vi "Mod_OFDM_Generate_Frame_per_Sub_Carrier.vi"(0 "Configure Variant":variant, 7 "Pool of Modulators":T3, 11 "error in":errorcluster, 12 "Pool of Data Sources":T2 {"Register Initial State" format="%08x"}, 13 "Symbol names in Frame":string[](array[string]), 14 "# of Symbols":i32) -> (4 "Parameters per OFDM Symbol":T1 {"Data Source"."Data Source"."Register Initial State" format="%08x"}, 15 "error out":errorcluster)   [LabVIEW 2010]
uses:
  Controls(Type_DEf)/Attribute Data Types.ctl
  Controls(Type_DEf)/Configure Pulse Shaping.ctl
  Controls(Type_DEf)/Pool of Modulator Control.ctl
  Controls(Type_DEf)/Pool of Data Source Control.ctl
  Controls(Type_DEf)/Attribute Names.ctl
  Controls(Type_DEf)/Parameters per Ofdm Symbol.ctl
panel:
  in  "Attribute Data Types":T4={"Pulse Shaping"={"System Filter"={"TX Filter"=enum."none", "Alpha"=0.0, "filter length"=0}, "Modulation system parameters"={"samples per symbol (16)"=0}, "symbol rate (Hz)"=0.0}, "FRAME Table"=[], "OFDM Frame"=[], "Sub Carrier Selection"={"Sub Carrier Selection"=[], "OFDM Parameters"={"# of Sub Carrier"=0, "Length Of Cylic Prefix"=0}}, "Symbol Table"=[], "Symbol Pool"=[], "Pool of Modulators"=[], "Pool of Data Sources"=[], "Atribute Names"={"Data Source Pool"="Data Source Pool ", "Modulator Source Pool"="Modulator Source Pool ", "OFDM SYMBOL POOL"="OFDM SYMBOL POOL", "Symbol Table"="Symbol Table", "Sub Carrier Selection"="Sub Carrier Selection", "OFDM Frame"="OFDM Frame", "FRAME Table"="FRAME Table", "Pulse Shaping"="Pulse Shaping"}} {"Pool of Data Sources"."Register Initial State" format="%08x"; "Pulse Shaping"."symbol rate (Hz)" min=1.0 step=1.0 format="%.2p"; "Pulse Shaping"."Modulation system parameters"."samples per symbol (16)" step=2; "Pulse Shaping"."System Filter"."Alpha" min=0.0 max=1.0 step=0.05 format="%.2f"}
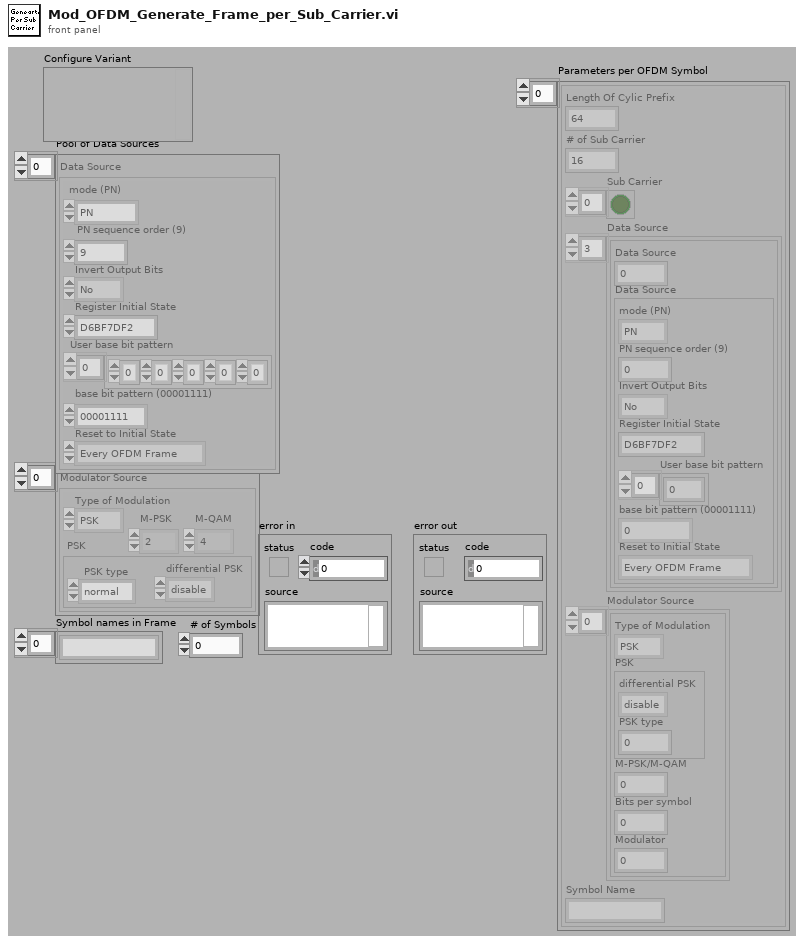
[diagram p1: front panel]
types:
  T1 = typedef "Parameters per Ofdm Symbol.ctl" = cluster{"Length Of Cylic Prefix":i32, "# of Sub Carrier":i32, "Sub Carrier":bool[], "Data Source":cluster{"Data Source":u16, "Data Source":cluster{"mode (PN)":enum16{"PN", "pattern", "user"}, "PN sequence order (9)":i32, "Invert Output Bits":enum16{"No", "Yes"}, "Register Initial State":u32, "User base bit pattern":i8[], "base bit pattern (00001111)":enum16{"0", "1", "01", "0011", "00001111"}, "Reset to Initial State":enum16{"Every OFDM Frame", "Every OFDM Symbol", "Every Sub Carrier"}}}[], "Modulator Source":cluster{"Type of Modulation":enum16{"PSK", "QAM"}, "PSK":cluster{"differential PSK":enum16{"disable", "enable"}, "PSK type":u16}, "M-PSK/M-QAM":i32, "Bits per symbol":i32, "Modulator":u16}[], "Symbol Name":string}[]
  T2 = typedef "Pool of Data Source Control.ctl" = cluster{"mode (PN)":enum16{"PN", "pattern", "user"}, "PN sequence order (9)":i32, "Invert Output Bits":enum16{"No", "Yes"}, "Register Initial State ":u32, "User base bit pattern":i8[], "base bit pattern (00001111)":enum16{"0", "1", "01", "0011", "00001111"}, "Reset to Initial State":enum16{"Every OFDM Frame", "Every OFDM Symbol", "Every Sub Carrier"}}[]
  T3 = typedef "Pool of Modulator Control.ctl" = cluster{"M-QAM":enum16{"4", "16", "64", "256"}, "M-PSK":enum16{"2", "4", "8", "16", "32", "64", "128", "256"}, "Type of Modulation":enum16{"PSK", "QAM"}, " PSK":cluster{"differential PSK":enum16{"disable", "enable"}, "PSK type":enum16{"normal", "shifted", "offset"}}}[]
  T4 = typedef "Attribute Data Types.ctl" = cluster{"Pulse Shaping":T5, "FRAME Table":string[][], "OFDM Frame":cluster{"Symbol Name":string, "# of Symbols":i32}[], "Sub Carrier Selection":cluster{"Sub Carrier Selection":cluster{"Sub Carrier":bool, "Data Source":u16, "Modulator":u16}[], "OFDM Parameters":cluster{"# of Sub Carrier":i32, "Length Of Cylic Prefix":i32}}, "Symbol Table":string[][], "Symbol Pool":string[], "Pool of Modulators":T3, "Pool of Data Sources":T2, "Atribute Names":T6}
  T5 = typedef "Configure Pulse Shaping.ctl" = cluster{"System Filter":cluster{"TX Filter":enum16{"none", "Raised Cosine", "Root Raised Cos"}, "Alpha":dbl, "filter length":i32}, "Modulation system parameters":cluster{"samples per symbol (16)":u32}, "symbol rate (Hz)":dbl}
  T6 = typedef "Attribute Names.ctl" = cluster{"Data Source Pool":string, "Modulator Source Pool":string, "OFDM SYMBOL POOL":string, "Symbol Table":string, "Sub Carrier Selection":string, "OFDM Frame":string, "FRAME Table":string, "Pulse Shaping":string}
  T7 = cluster{"Type of Modulation":enum16{"PSK", "QAM"}, "PSK":cluster{"differential PSK":enum16{"disable", "enable"}, "PSK type":u16}, "M-PSK/M-QAM":i32, "Bits per symbol":i32, "Modulator":u16}
  T8 = cluster{"Sub Carrier Selection":cluster{"Sub Carrier":bool, "Data Source":u16, "Modulator":u16}[], "OFDM Parameters":cluster{"# of Sub Carrier":i32, "Length Of Cylic Prefix":i32}}
  T9 = cluster{"Sub Carrier":bool, "Data Source":u16, "Modulator":u16}[]
  T10 = cluster{"Sub Carrier":bool, "Data Source":u16, "Modulator":u16}
  T11 = cluster{"mode (PN)":enum16{"PN", "pattern", "user"}, "PN sequence order (9)":i32, "Invert Output Bits":enum16{"No", "Yes"}, "Register Initial State ":u32, "User base bit pattern":i8[], "base bit pattern (00001111)":enum16{"0", "1", "01", "0011", "00001111"}, "Reset to Initial State":enum16{"Every OFDM Frame", "Every OFDM Symbol", "Every Sub Carrier"}}
  T12 = cluster{"M-QAM":enum16{"4", "16", "64", "256"}, "M-PSK":enum16{"2", "4", "8", "16", "32", "64", "128", "256"}, "Type of Modulation":enum16{"PSK", "QAM"}, " PSK":cluster{"differential PSK":enum16{"disable", "enable"}, "PSK type":enum16{"normal", "shifted", "offset"}}}
  T13 = enum16{"2", "4", "8", "16", "32", "64", "128", "256"}
  T14 = cluster{"differential PSK":enum16{"disable", "enable"}, "PSK type":enum16{"normal", "shifted", "offset"}}
  T15 = cluster{"Data Source":u16, "Data Source":cluster{"mode (PN)":enum16{"PN", "pattern", "user"}, "PN sequence order (9)":i32, "Invert Output Bits":enum16{"No", "Yes"}, "Register Initial State ":u32, "User base bit pattern":i8[], "base bit pattern (00001111)":enum16{"0", "1", "01", "0011", "00001111"}, "Reset to Initial State":enum16{"Every OFDM Frame", "Every OFDM Symbol", "Every Sub Carrier"}}}
  T16 = cluster{"Length Of Cylic Prefix":i32, "# of Sub Carrier":i32, "Sub Carrier":bool[], "Data Source":cluster{"Data Source":u16, "Data Source":cluster{"mode (PN)":enum16{"PN", "pattern", "user"}, "PN sequence order (9)":i32, "Invert Output Bits":enum16{"No", "Yes"}, "Register Initial State":u32, "User base bit pattern":i8[], "base bit pattern (00001111)":enum16{"0", "1", "01", "0011", "00001111"}, "Reset to Initial State":enum16{"Every OFDM Frame", "Every OFDM Symbol", "Every Sub Carrier"}}}[], "Modulator Source":cluster{"Type of Modulation":enum16{"PSK", "QAM"}, "PSK":cluster{"differential PSK":enum16{"disable", "enable"}, "PSK type":u16}, "M-PSK/M-QAM":i32, "Bits per symbol":i32, "Modulator":u16}[], "Symbol Name":string}
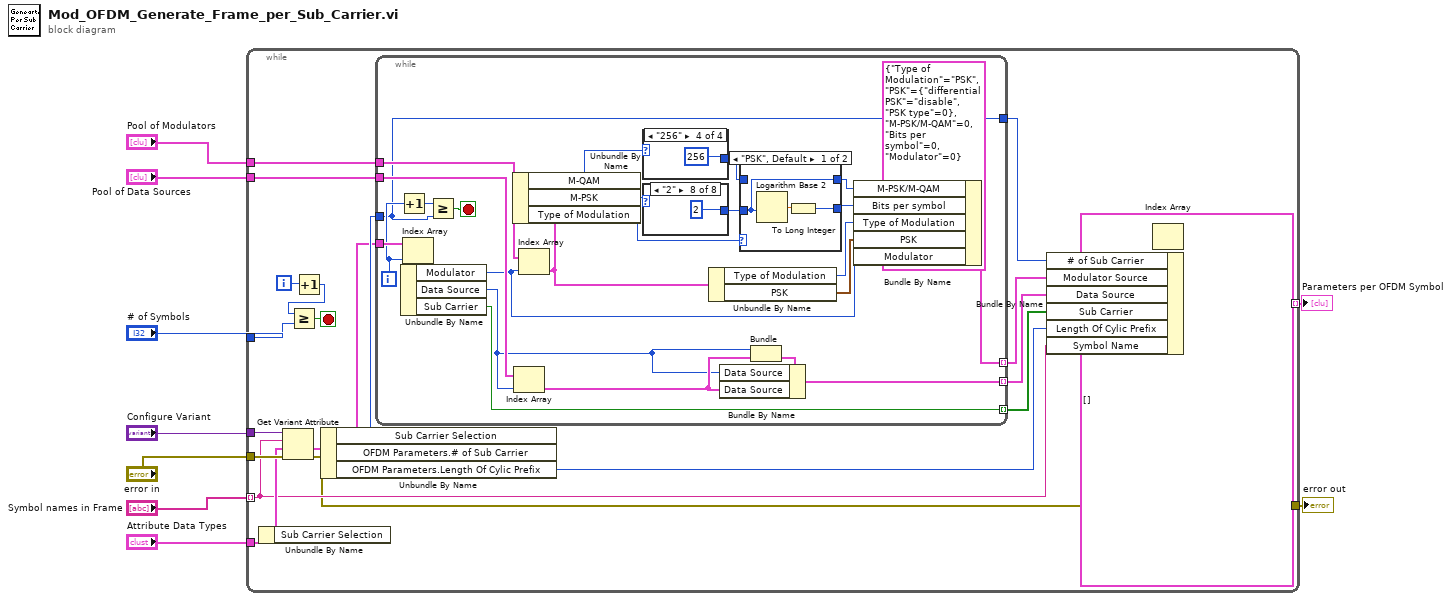
[diagram p0: block diagram]
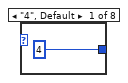
[diagram p2: hidden frame]
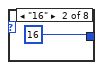
[diagram p3: hidden frame]
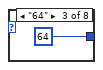
[diagram p4: hidden frame]
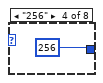
[diagram p5: hidden frame]
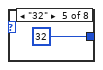
[diagram p6: hidden frame]
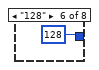
[diagram p7: hidden frame]
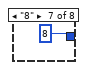
[diagram p8: hidden frame]
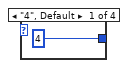
[diagram p9: hidden frame]
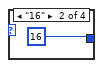
[diagram p10: hidden frame]
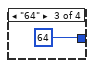
[diagram p11: hidden frame]
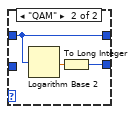
[diagram p12: hidden frame]
diagram:
  n1 = while {
    tunnel: "Pool of Data Sources" -> [w32]
    tunnel: "Pool of Modulators" -> [w31]
    tunnel: "Symbol names in Frame" -> [w18] mode=indexing
    tunnel: "Configure Variant" -> [w28]
    tunnel: "# of Symbols" -> [w24]
    tunnel: [w12] -> w4
    tunnel: "Attribute Data Types" -> [w22]
    tunnel: "error in" -> [w23]
    tunnel: [w19] -> w1 mode=indexing
    i -> [w27]
    stop <- w25 stop-if-true
    n2 = Unbundle By Name(w22) -> ("Sub Carrier Selection"=w21:T8)
    n3 = Get Variant Attribute(Variant=w28, name=w18, default value (empty Variant)=w21, error in=w23) -> (value=w20:T8, error out=w12:errorcluster)  [unwired: 2 out]
    n4 = Increment(x=w27) -> (x+1=w26:i32)
    n5 = Greater Or Equal?(x=w26, y=w24) -> (x >= y?=w25:bool)
    n6 = Unbundle By Name(w20) -> ("Sub Carrier Selection"=w29:T9, "OFDM Parameters.# of Sub Carrier"=w30:i32, "OFDM Parameters.Length Of Cylic Prefix"=w17:i32)
    n7 = while {
      tunnel: w29 -> [w58]
      tunnel: w30 -> [w45]
      tunnel: [w53] -> w16 mode=indexing
      tunnel: w31 -> [w52]
      tunnel: w32 -> [w51]
      tunnel: [w45] -> w14
      tunnel: [w40] -> w15 mode=indexing
      tunnel: [w38] -> w13 mode=indexing
      i -> [w57]
      stop <- w55 stop-if-true
      n8 = Increment(x=w57) -> (x+1=w56:i32)
      n9 = Index Array(array=w58, index=w57) -> (element=w54:T10)
      n10 = Unbundle By Name(w54) -> ("Modulator"=w36:u16, "Data Source"=w34:u16, "Sub Carrier"=w53:bool)
      n11 = Greater Or Equal?(x=w56, y=w45) -> (x >= y?=w55:bool)
      n12 = Index Array(array=w51, index=w34) -> (element=w35:T11)
      n13 = Index Array(array=w52, index=w36) -> (element=w37:T12)
      n14 = Unbundle By Name(w37) -> ("M-QAM"=w49:enum16{"4", "16", "64", "256"}, "M-PSK"=w48:T13, "Type of Modulation"=w50:enum16{"PSK", "QAM"})
      n15 = case shown="\"256\"" w49 {
        tunnel: [4 16 64 256] -> w46
        frame "4", Default {
        }
        frame "16" {
        }
        frame "64" {
        }
        frame "256" {
        }
      }
      n16 = case shown="\"2\"" w48 {
        tunnel: [4 16 64 256 32 128 8 2] -> w47
        frame "4", Default {
        }
        frame "16" {
        }
        frame "64" {
        }
        frame "256" {
        }
        frame "32" {
        }
        frame "128" {
        }
        frame "8" {
        }
        frame "2" {
        }
      }
      n17 = Unbundle By Name(w37) -> ("Type of Modulation"=w43:enum16{"PSK", "QAM"}, "PSK"=w44:T14)
      n18 = case shown="\"PSK\", Default" w50 {
        tunnel: w47 -> [w71 _]
        tunnel: w46 -> [_ w74]
        tunnel: [w72 w76] -> w42
        tunnel: [w71 w74] -> w41
        frame "PSK", Default {
          n19 = Logarithm Base 2(1:w71) -> (0:w73:dbl)
          n20 = To Long Integer(number=w73) -> (32bit integer=w72:i32)
        }
        frame "QAM" {
          n21 = Logarithm Base 2(1:w74) -> (0:w75:dbl)
          n22 = To Long Integer(number=w75) -> (32bit integer=w76:i32)
        }
      }
      n23 = Bundle("Data Source"=w34, "Data Source"=w35) -> (w33:T15)  [unwired: 1 in]
      n24 = Bundle By Name(cluster=w33, "Data Source"=w34, "Data Source"=w35) -> (w38:T15)
      n25 = Bundle By Name(cluster=T7 {"Type of Modulation"=enum."PSK", "PSK"={"differential PSK"=enum."disable", "PSK type"=0}, "M-PSK/M-QAM"=0, "Bits per symbol"=0, "Modulator"=0} ("element"), "M-PSK/M-QAM"=w41, "Bits per symbol"=w42, "Type of Modulation"=w43, "PSK"=w44, "Modulator"=w36) -> (w40:T7)
    }
    n26 = Index Array(array=T1 [] ("Parameters per Ofdm Symbol")) -> (element=w10:T16)  [unwired: 1 in]
    n27 = Bundle By Name(cluster=w10, "# of Sub Carrier"=w14, "Modulator Source"=w15, "Data Source"=w13, "Sub Carrier"=w16, "Length Of Cylic Prefix"=w17, "Symbol Name"=w18) -> (w19:T16)
  }
  "error out" <- w4
  "Parameters per OFDM Symbol" <- w1
